vi "SUB_NI_Close_COM6.vi"() -> (0 "error":i32)   [LabVIEW 2011]
doc: "Closes the specified port."
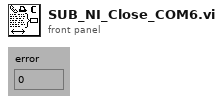
[diagram p1: front panel]
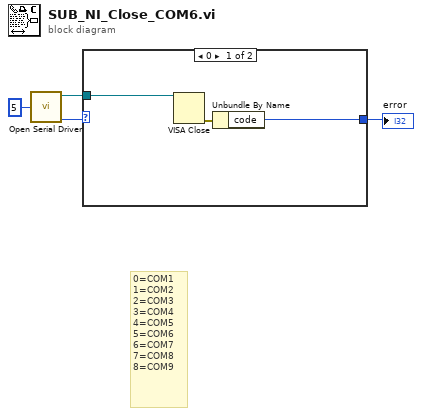
[diagram p0: block diagram]
diagram:
  # "0=COM1\n1=COM2\n2=COM3\n3=COM4\n4=COM5\n5=COM6\n6=COM7\n7=COM8\n8=COM9"
  n1 = call <vilib>:"Open Serial Driver.vi"("port number"=u32 5) -> ("input refnum"=w3:refnum<visa-resource-name>, "output error"=w4:i32)  [unwired: 2 out]
  n2 = case shown="0" w4 {
    selector: w4 -> [_ w8]
    tunnel: w3 -> [w7 _]
    tunnel: [w5 w8] -> w2
    frame 0 {
      n3 = VISA Close(VISA resource name=w7) -> (error out=w6:errorcluster)  [unwired: 1 in]
      n4 = Unbundle By Name(w6) -> ("code"=w5:i32)
    }
    frame 1, Default {
    }
  }
  "error" <- w2
